vi "Initiallize EMG Task.vi"(7 "TDMS File":refnum<k34>, 8 "error in (no error)":errorcluster, 9 "EMG Master Config":T1, 10 "EMG info":cluster{"Collect EMG?":bool, "EMG Rate":u16}, 11 "NI Force Task in":refnum<class "NI Force Task.lvclass">) -> (0 "error out":errorcluster, 3 "NI Force Task out":refnum<class "NI Force Task.lvclass">)   [LabVIEW 2020, in "NI Force Task.lvlib" / "NI Force Task.lvclass"]
uses:
  NI Force Task.lvclass
  EMG channels df.ctl
  NI Force Task.lvclass/NI Force Task.ctl
  <vilib>/DAQmx/create/channels.llb/DAQmx Create Channel (AI-Voltage-Basic).vi
  <vilib>/DAQmx/configure/timing.llb/DAQmx Timing (Sample Clock).vi
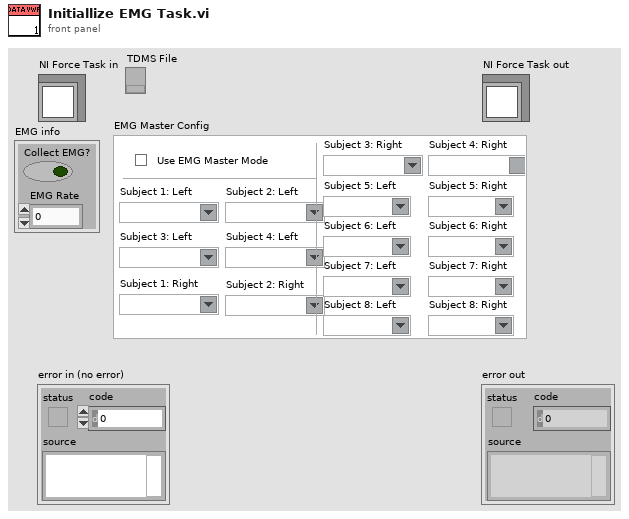
[diagram p1: front panel]
types:
  T1 = typedef "EMG channels df.ctl" = cluster{"EMG Master":bool, "EMGL1":tag, "EMGR1":tag, "EMGL2":tag, "EMGR2":tag, "EMGL3":tag, "EMGR3":tag, "EMGL4":tag, "EMGR4":tag, "EMGL5":tag, "EMGR5":tag, "EMGL6":tag, "EMGR6":tag, "EMGL7":tag, "EMGR7":tag, "EMGL8":tag, "EMGR8":tag}
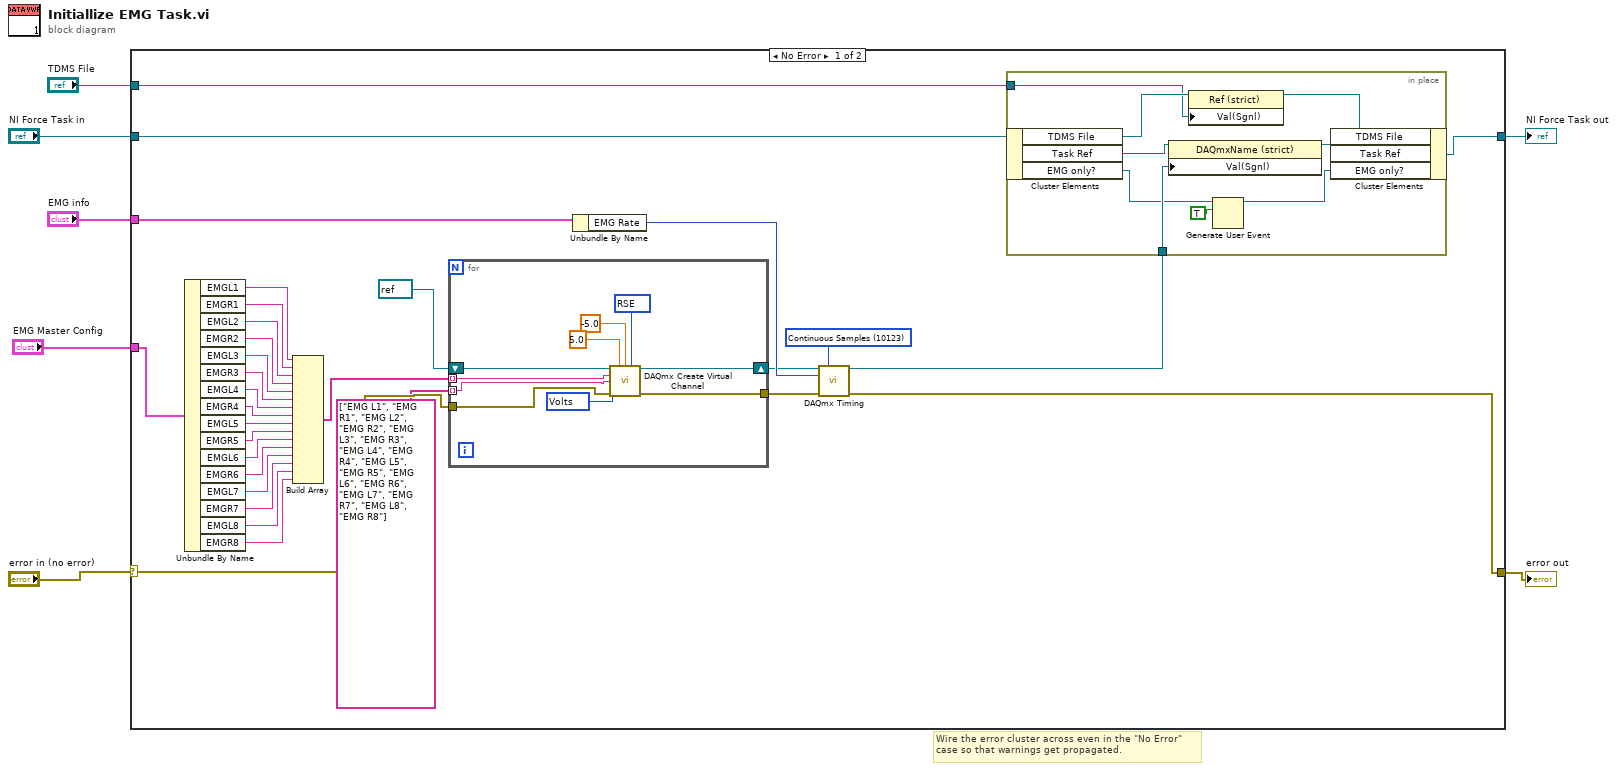
[diagram p0: block diagram]
diagram:
  # "Wire the error cluster across even in the \"No Error\"\ncase so that warnings get propagated."
  n1 = case shown="No Error" "error in (no error)" {
    selector: "error in (no error)" -> [w18 w59]
    tunnel: [w21 w59] -> w6
    tunnel: [w24 w58] -> w4
    tunnel: "NI Force Task in" -> [w25 w58]
    tunnel: "EMG Master Config" -> [w38 _]
    tunnel: "EMG info" -> [w27 _]
    tunnel: "TDMS File" -> [w23 _]
    frame No Error {
      w29 = 10123 items=["Finite Samples"=10178, "Continuous Samples"=10123, "Hardware Timed Single Point"=12522] ("sample mode")
      n2 = Unbundle By Name(w38) -> ("EMGL1"=w37:tag, "EMGR1"=w36:tag, "EMGL2"=w35:tag, "EMGR2"=w34:tag, "EMGL3"=w33:tag, "EMGR3"=w32:tag, "EMGL4"=w31:tag, "EMGR4"=w30:tag, "EMGL5"=w15:tag, "EMGR5"=w14:tag, "EMGL6"=w13:tag, "EMGR6"=w12:tag, "EMGL7"=w11:tag, "EMGR7"=w10:tag, "EMGL8"=w9:tag, "EMGR8"=w8:tag)
      n3 = Build Array(w37, w36, w35, w34, w33, w32, w31, w30, w15, w14, w13, w12, w11, w10, w9, w8) -> (w19:tag[])
      n4 = for {
        tunnel: [w43] -> w28
        tunnel: w19 -> [w41] mode=indexing
        shift-right: [w44] -> w16
        shift-left: refnum<k21> refnum ("task in") -> [w42]
        tunnel: w18 -> [w40]
        tunnel: string[] ["EMG L1", "EMG R1", "EMG L2", "EMG R2", "EMG L3", "EMG R3", "EMG L4", "EMG R4", "EMG L5", "EMG R5", "EMG L6", "EMG R6", "EMG L7", "EMG R7", "EMG L8", "EMG R8"] -> [w39] mode=indexing
        w45 = 10348 items=["Volts"=10348, "From Custom Scale"=10065] ("units")
        w48 = 10083 items=["Default"=-1, "RSE"=10083, "NRSE"=10078, "Differential"=10106, "Pseudodifferential"=12529] ("input terminal configuration")
        n5 = call-poly <vilib>:"DAQmx Create Virtual Channel.vi"("task in"=w42, "maximum value"=5.0, "minimum value"=-5.0, "input terminal configuration"=w48, "physical channels"=w41, "name to assign"=w39, "units"=w45, "error in"=w40) -> ("task out"=w44:refnum<k21>, "error out"=w43:errorcluster)  [unwired: 6 in]
      }
      n6 = Unbundle By Name(w27) -> ("EMG Rate"=w26:u16)
      n7 = call-poly <vilib>:"DAQmx Timing.vi"("task/channels in"=w16, "sample mode"=w29, "rate"=w26, "error in"=w28) -> ("task out"=w22:refnum<k21>, "error out"=w21:errorcluster)  [unwired: 10 in]
      n8 = in-place {
        in-place-border: w23 -> [w55]
        in-place-border: w22 -> [w52]
        n9 = in-place-cluster #1(w25) -> ("TDMS File"=w56:refnum<vi>, "Task Ref"=w57:refnum<vi>, "EMG only?"=w51:refnum<user-event>)
        n10 = property class="DAQmxName (strict)"(reference=w57, "Val(Sgnl)"=w52) -> (reference out=w54:refnum<vi>)  [unwired: 1 in, 1 out]
        n11 = property class="Ref (strict)"(reference=w56, "Val(Sgnl)"=w55) -> (reference out=w53:refnum<vi>)  [unwired: 1 in, 1 out]
        n12 = Generate User Event(user event=w51, event data cluster=TRUE ("Value (Signaling)")) -> (user event out=w49:refnum<user-event>)  [unwired: 2 in, 1 out]
        n13 = in-place-cluster #1("TDMS File"=w53, "Task Ref"=w54, "EMG only?"=w49) -> (w24:refnum<class "NI Force Task.lvclass">)
      }
    }
    frame Error {
    }
  }
  "error out" <- w6
  "NI Force Task out" <- w4
